vi "Write Metrics.vi"(8 "error in (no error)":errorcluster, 10 "Metrics":refnum<data-value>[](array[refnum]), 11 "Default Collector in":refnum<class "Default Collector.lvclass">) -> (0 "error out":errorcluster, 3 "Default Collector out":refnum<class "Default Collector.lvclass">)   [LabVIEW 2020, in "Collector.lvlib" / "Default Collector.lvclass"]
uses:
  Default Collector.lvclass
  metrics/metric/Metric.lvclass
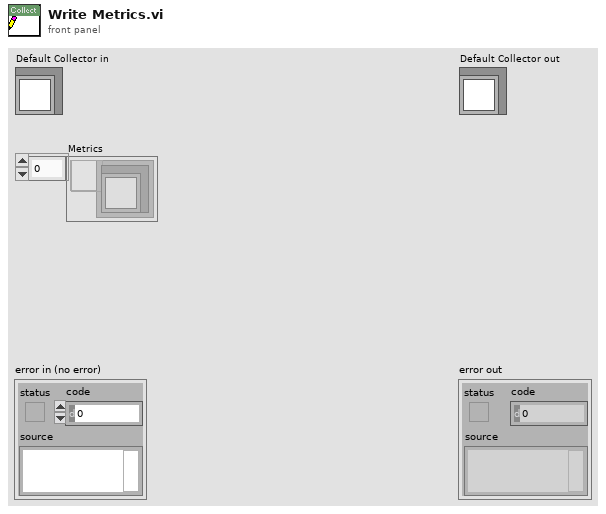
[diagram p1: front panel]
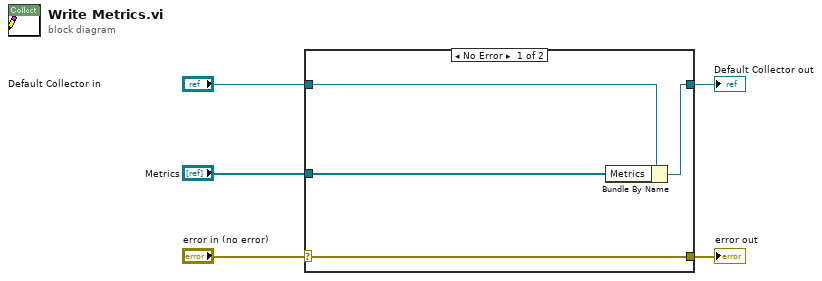
[diagram p0: block diagram]
diagram:
  n1 = case shown="No Error" "error in (no error)" {
    selector: "error in (no error)" -> [w9 w10]
    tunnel: [w9 w10] -> w4
    tunnel: [w7 w11] -> w2
    tunnel: "Default Collector in" -> [w8 w11]
    tunnel: "Metrics" -> [w6 _]
    frame No Error {
      n2 = Bundle By Name(cluster=w8, "Metrics"=w6) -> (w7:refnum<class "Default Collector.lvclass">)
    }
    frame Error {
    }
  }
  "error out" <- w4
  "Default Collector out" <- w2
